vi "Activity Light - Exit.vi"(8 "error in (no error)":errorcluster, 11 "Name":string="Activity Light") -> (0 "error out":errorcluster)   [LabVIEW 2024, in "EQMF.lvlib" / "Status Utils.lvlib"]
uses:
  Status Utils.lvlib
  _Private/Activity Light Q Item.ctl
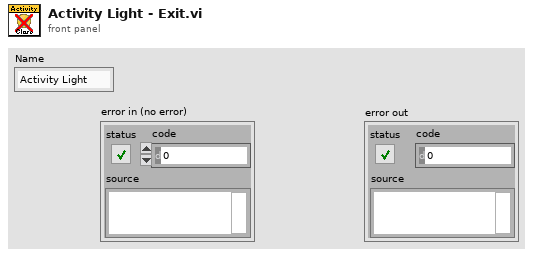
[diagram p1: front panel]
types:
  T1 = typedef "EQMF.lvlib/Status Utils.lvlib/Activity Light Q Item.ctl" = cluster{"Cmd":string, "Data":variant}
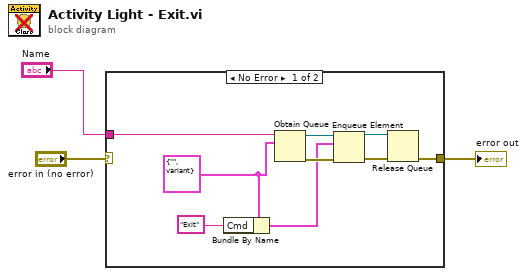
[diagram p0: block diagram]
diagram:
  n1 = case shown="No Error" "error in (no error)" {
    selector: "error in (no error)" -> [_ w13]
    tunnel: [w8 w13] -> w3
    tunnel: "Name" -> [w4 _]
    frame No Error {
      w7 = T1 {"Cmd"="", "Data"=variant} ("output cluster")
      n2 = Bundle By Name(cluster=w7, "Cmd"="Exit") -> (w6:T1)
      n3 = Obtain Queue(name (unnamed)=w4, element data type=w7) -> (queue out=w12:refnum<queue>, error out=w11:errorcluster)  [unwired: 3 in, 1 out]
      n4 = Enqueue Element(queue=w12, element=w6, error in (no error)=w11) -> (queue out=w9:refnum<queue>, error out=w10:errorcluster)  [unwired: 1 in, 1 out]
      n5 = Release Queue(queue=w9, error in (no error)=w10) -> (error out=w8:errorcluster)  [unwired: 1 in, 2 out]
    }
    frame Error {
    }
  }
  "error out" <- w3
